vi "ON_ALIM-Wkup.vi"(8 "errin":errorcluster, 11 "VISA J1":refnum<visa-resource-name>) -> (0 "errout":errorcluster)   [LabVIEW 2020]
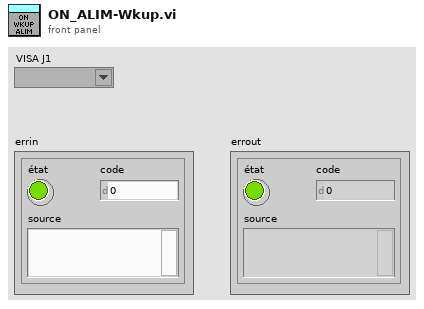
[diagram p1: front panel]
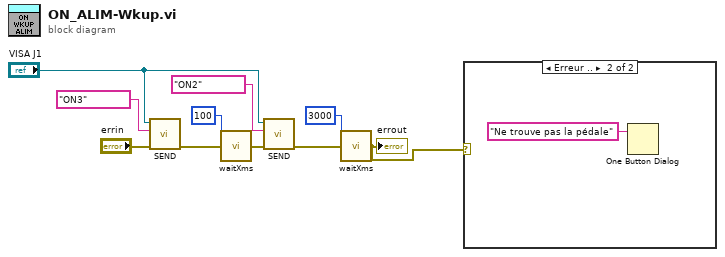
[diagram p0: block diagram]
diagram:
  n1 = call "SEND.vi"("errin"="errin", "chaîne"="ON3" ("CMD"), "visa in"="VISA J1") -> ("errout"=w8:errorcluster)  [unwired: 6 in, 2 out]
  n2 = call "waitXms.vi"("attente (ms)"=u32 100, "errin"=w8) -> ("errout"=w6:errorcluster)  [unwired: 13 in]
  n3 = call "SEND.vi"("errin"=w6, "chaîne"="ON2" ("CMD"), "visa in"="VISA J1") -> ("errout"=w4:errorcluster)  [unwired: 6 in, 2 out]
  n4 = call "waitXms.vi"("attente (ms)"=u32 3000, "errin"=w4) -> ("errout"=w1:errorcluster)  [unwired: 13 in]
  "errout" <- w1
  n5 = case shown="Erreur .." w1 {
    frame No Error {
    }
    frame Error {
      n6 = One Button Dialog(message="Ne trouve pas la pédale") -> ()  [unwired: 1 in, 1 out]
    }
  }
